vi "uc480_ArrayToImage.vi"(8 "Error In":errorcluster, 10 "InArray":u8[](array[numeric]), 11 ".NET (Reference)":refnum<k24>) -> (0 "Error Out":errorcluster, 2 "Image":picture, 3 "Image Out":T1(plugin-control))   [LabVIEW 2015]
doc: "ArrayToVision converts 24/32-bit one-dimensional arrays to a two-dimensional U32 array."
uses:
  C:/Program Files/Thorlabs/Scientific Imaging/DCx Camera Support/Develop/DotNet/uc480DotNet.dll
  <vilib>/picture/picture.llb/Draw True-Color Pixmap.vi
panel:
  out "SensorColorMode":i32(ring) items=["Invalid"=0, "Monochrome"=1, "Bayer"=2, "CBYCRY"=4, "Jpeg"=8]
  out "Numeric":i32
  # "Input"
  # "Output"
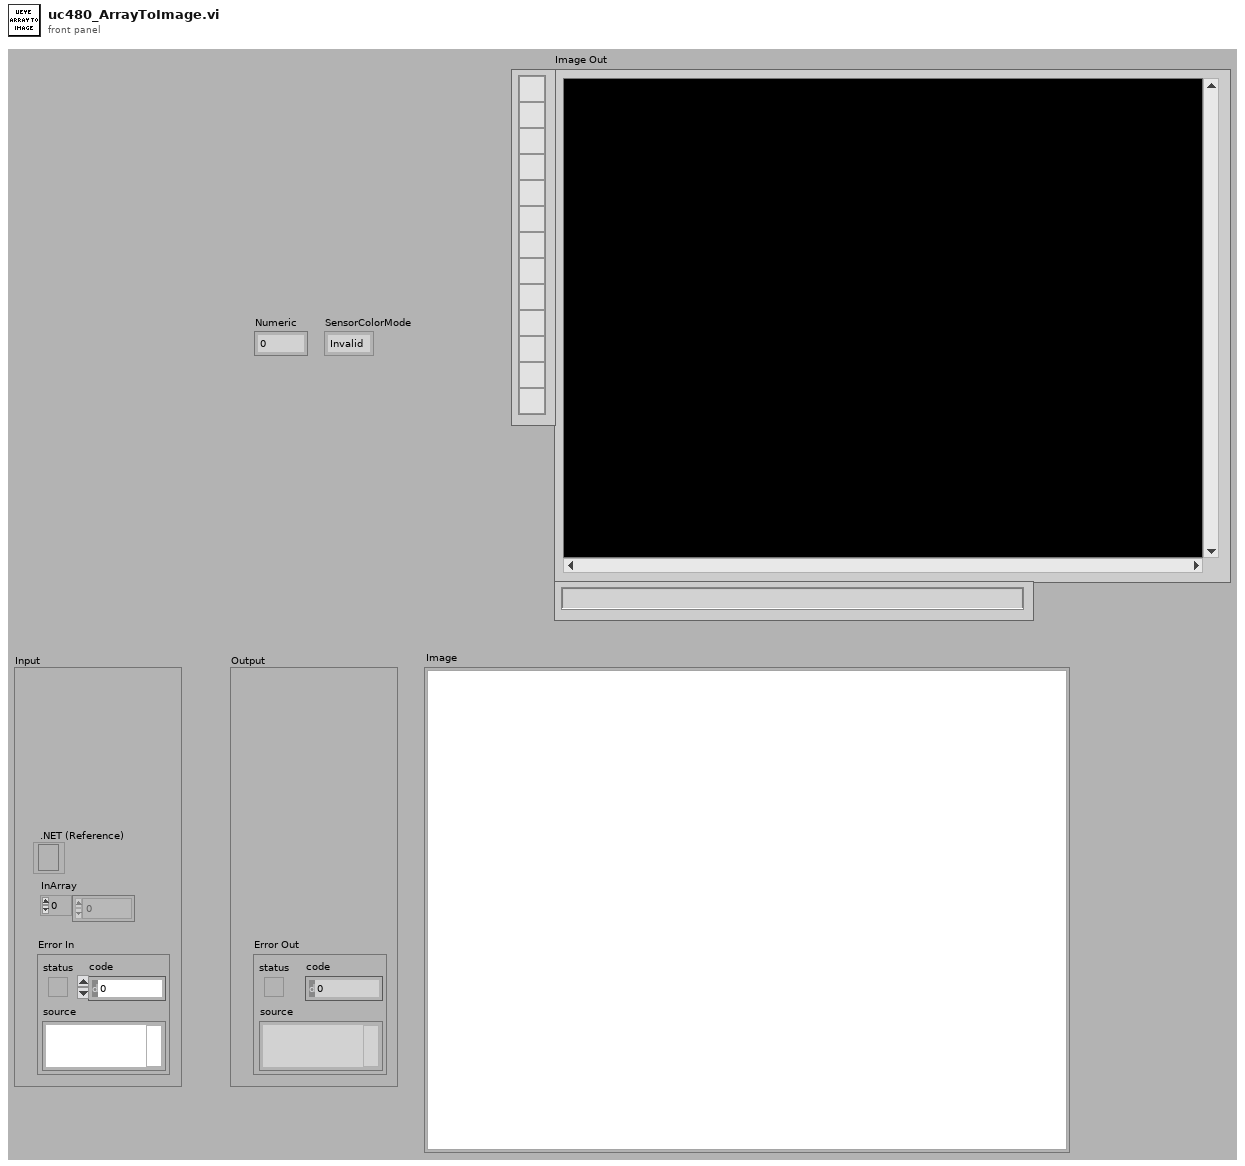
[diagram p1: front panel]
types:
  T1 = typedef "IMAQ Image.ctl" = refnum<image>
  T2 = typedef "Image Type" = u32
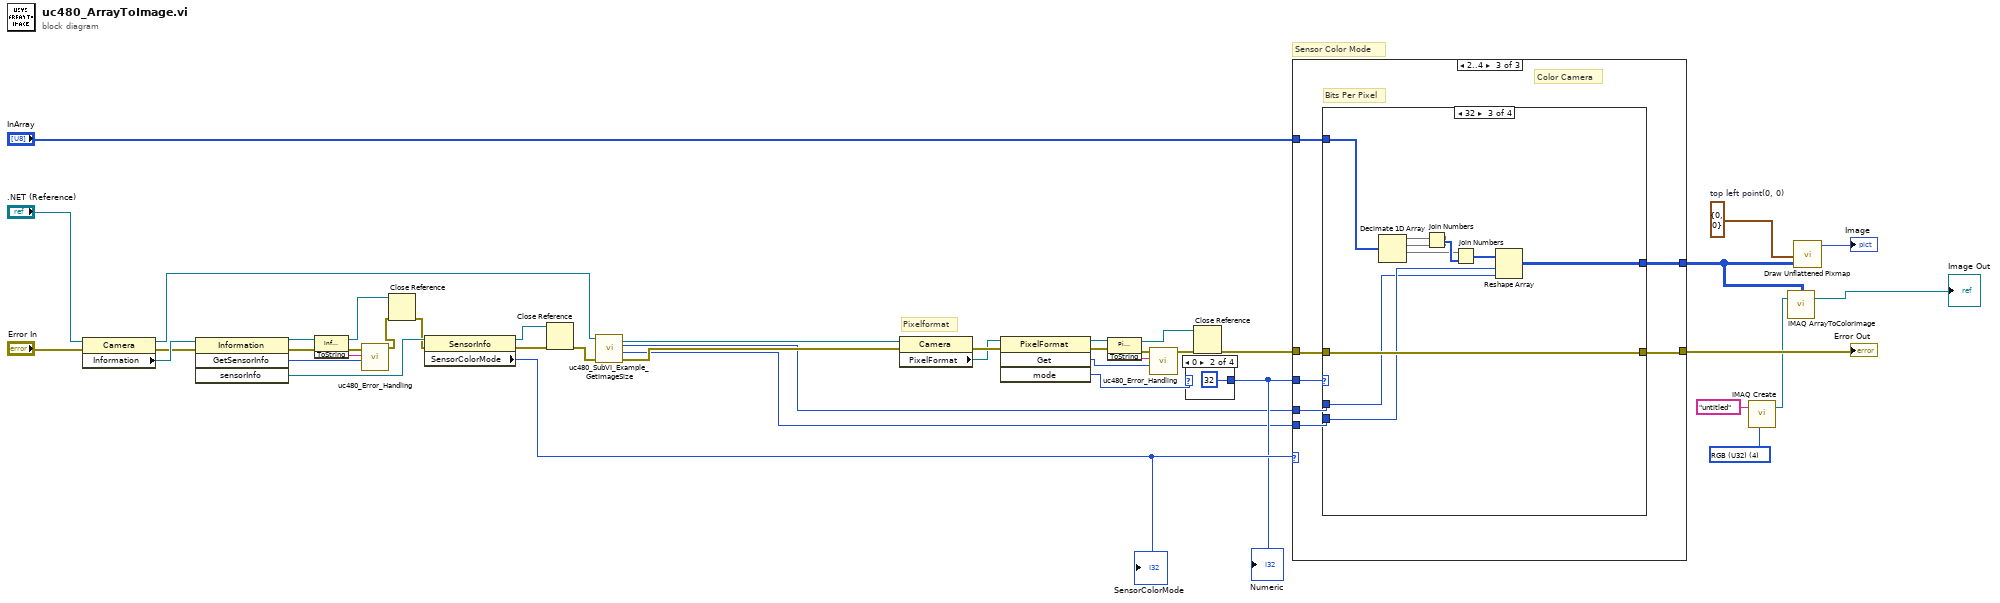
[diagram p0: block diagram]
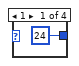
[diagram p2: hidden frame]
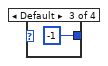
[diagram p3: hidden frame]
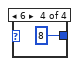
[diagram p4: hidden frame]
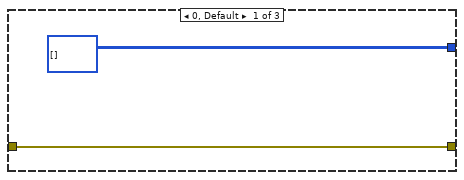
[diagram p5: hidden frame]
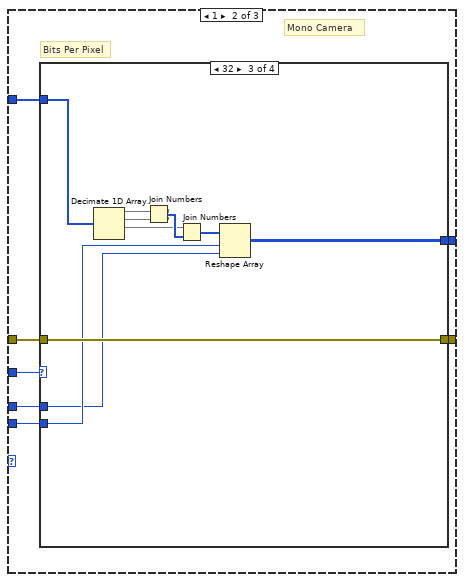
[diagram p6: hidden frame]
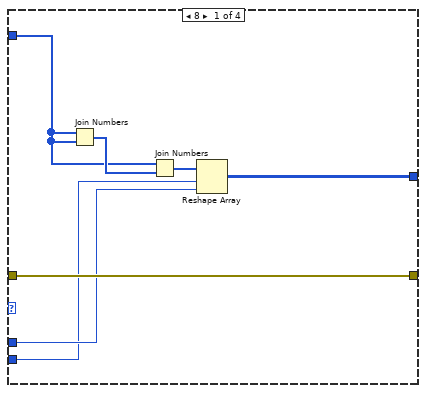
[diagram p7: hidden frame]
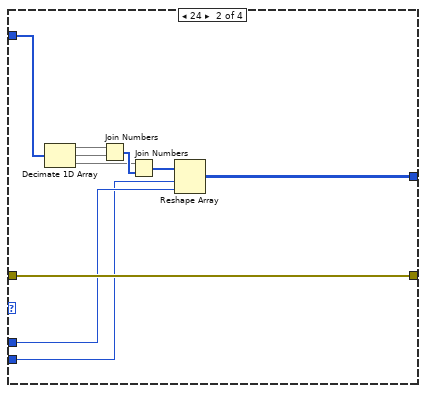
[diagram p8: hidden frame]
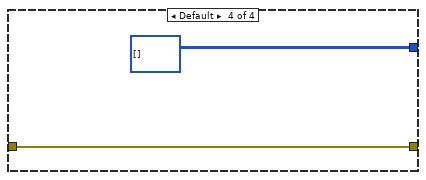
[diagram p9: hidden frame]
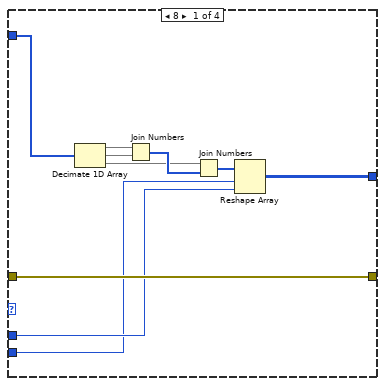
[diagram p10: hidden frame]
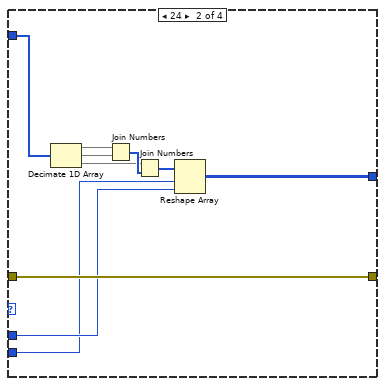
[diagram p11: hidden frame]
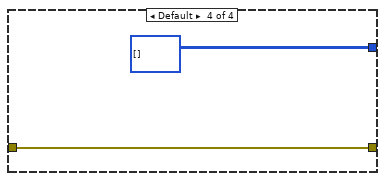
[diagram p12: hidden frame]
diagram:
  w2 = T2 4 items=["Grayscale (U8)", "Grayscale (I16)", "Grayscale (SGL)", "Complex (CSG)", "RGB (U32)", "HSL (U32)", "RGB (U64)", "Grayscale (U16)"] ("Image Type")
  w43 = cluster{i16, i16} {0, 0}  # top left point(0, 0)
  # "Sensor Color Mode"
  # "Pixelformat"
  n1 = property on="Eigenschaftsknoten" class="Camera"(reference=".NET (Reference)", error in="Error In") -> (reference out=w6:refnum<k24>, error out=w38:errorcluster, "Information"=w41:refnum<k24>)
  n2 = invoke class="Information" method="GetSensorInfo"(reference=w41, error in=w38) -> (reference out=w33:refnum<k24>, error out=w32:errorcluster, "GetSensorInfo"=w31:i32, "sensorInfo"=w40:refnum<k24>)  [unwired: 2 in]
  n3 = invoke class="Information" method="ToString"(reference=w33, error in=w32) -> (reference out=w15:refnum<k24>, error out=w35:errorcluster, "ToString"=w34:string)  [unwired: 1 in]
  n4 = call "uc480_Error_Handling.vi"("Error Code"=w31, "Error String"=w34, "Error In"=w35) -> ("Error Out"=w14:errorcluster)  [unwired: 8 in]
  n5 = Close Reference(reference=w15, error in (no error)=w14) -> (error out=w13:errorcluster)
  n6 = property class="SensorInfo"(reference=w40, error in=w13) -> (reference out=w12:refnum<k24>, error out=w11:errorcluster, "SensorColorMode"=w39:i32)
  "SensorColorMode" <- w39
  n7 = Close Reference(reference=w12, error in (no error)=w11) -> (error out=w10:errorcluster)
  n8 = call "uc480_SubVI_Example_GetImageSize.vi"("Error In"=w10, ".NET (Reference)"=w6) -> ("Error Out"=w20:errorcluster, "Height"=w16:i32, "Width"=w17:i32, ".NET (Reference)"=w18:refnum<k24>)  [unwired: 6 in]
  n9 = property class="Camera"(reference=w18, error in=w20) -> (error out=w25:errorcluster, "PixelFormat"=w24:refnum<k24>)  [unwired: 1 out]
  n10 = invoke class="PixelFormat" method="Get"(reference=w24, error in=w25) -> (reference out=w30:refnum<k24>, error out=w29:errorcluster, "Get"=w28:i32, "mode"=w23:i32)  [unwired: 2 in]
  n11 = invoke class="PixelFormat" method="ToString"(reference=w30, error in=w29) -> (reference out=w9:refnum<k24>, error out=w26:errorcluster, "ToString"=w27:string)  [unwired: 1 in]
  n12 = call "uc480_Error_Handling.vi"("Error Code"=w28, "Error String"=w27, "Error In"=w26) -> ("Error Out"=w8:errorcluster)  [unwired: 8 in]
  n13 = case shown="0" w23 {
    tunnel: [24 32 -1 8] -> w22
    frame 1 {
    }
    frame 0 {
    }
    frame Default {
    }
    frame 6 {
    }
  }
  "Numeric" <- w22
  n14 = Close Reference(reference=w9, error in (no error)=w8) -> (error out=w7:errorcluster)
  n15 = case shown="2..4" w39 {
    tunnel: "InArray" -> [_ w53 w92]
    tunnel: w17 -> [_ w51 w87]
    tunnel: w16 -> [_ w50 w86]
    tunnel: w22 -> [_ w52 w88]
    tunnel: w7 -> [w48 w56 w89]
    tunnel: [w48 w55 w90] -> w21
    tunnel: [u32[][] [] w54 w91] -> w1
    frame 0, Default {
    }
    frame 1 {
      # "Bits Per Pixel"
      # "Mono Camera"
      n16 = case shown="32" w52 {
        tunnel: w53 -> [w59 w68 w79 _]
        tunnel: w50 -> [w57 w64 w75 _]
        tunnel: w51 -> [w58 w65 w74 _]
        tunnel: [w63 w67 w81 u32[][] []] -> w54
        tunnel: w56 -> [w62 w66 w80 w84]
        tunnel: [w62 w66 w80 w84] -> w55
        frame 8 {
          n17 = Join Numbers(hi=w59, lo=w59) -> ((hi.lo)=w61:u16[])
          n18 = Join Numbers(hi=w59, lo=w61) -> ((hi.lo)=w60:u32[])
          n19 = Reshape Array(w60, w57, w58) -> (w63:u32[][])
        }
        frame 24 {
          n20 = Decimate 1D Array(w68) -> (w73:u8[], w72:u8[], w70:u8[])
          n21 = Join Numbers(hi=w72, lo=w73) -> ((hi.lo)=w71:u16[])
          n22 = Join Numbers(hi=w70, lo=w71) -> ((hi.lo)=w69:u32[])
          n23 = Reshape Array(w69, w64, w65) -> (w67:u32[][])
        }
        frame 32 {
          n24 = Decimate 1D Array(w79) -> (w78:u8[], w77:u8[], w76:u8[])  [unwired: 1 out]
          n25 = Join Numbers(hi=w77, lo=w78) -> ((hi.lo)=w83:u16[])
          n26 = Join Numbers(hi=w76, lo=w83) -> ((hi.lo)=w82:u32[])
          n27 = Reshape Array(w82, w75, w74) -> (w81:u32[][])
        }
        frame Default {
        }
      }
    }
    frame 2..4 {
      # "Bits Per Pixel"
      # "Color Camera"
      n28 = case shown="32" w88 {
        tunnel: w92 -> [w94 w107 w119 _]
        tunnel: w86 -> [w99 w103 w114 _]
        tunnel: w87 -> [w100 w104 w113 _]
        tunnel: [w102 w106 w120 u32[][] []] -> w91
        tunnel: w89 -> [w101 w105 w118 w123]
        tunnel: [w101 w105 w118 w123] -> w90
        frame 8 {
          n29 = Decimate 1D Array(w94) -> (w98:u8[], w97:u8[], w95:u8[])
          n30 = Join Numbers(hi=w97, lo=w98) -> ((hi.lo)=w96:u16[])
          n31 = Join Numbers(hi=w95, lo=w96) -> ((hi.lo)=w93:u32[])
          n32 = Reshape Array(w93, w99, w100) -> (w102:u32[][])
        }
        frame 24 {
          n33 = Decimate 1D Array(w107) -> (w112:u8[], w111:u8[], w109:u8[])
          n34 = Join Numbers(hi=w111, lo=w112) -> ((hi.lo)=w110:u16[])
          n35 = Join Numbers(hi=w109, lo=w110) -> ((hi.lo)=w108:u32[])
          n36 = Reshape Array(w108, w103, w104) -> (w106:u32[][])
        }
        frame 32 {
          n37 = Decimate 1D Array(w119) -> (w117:u8[], w116:u8[], w115:u8[])  [unwired: 1 out]
          n38 = Join Numbers(hi=w116, lo=w117) -> ((hi.lo)=w122:u16[])
          n39 = Join Numbers(hi=w115, lo=w122) -> ((hi.lo)=w121:u32[])
          n40 = Reshape Array(w121, w114, w113) -> (w120:u32[][])
        }
        frame Default {
        }
      }
    }
  }
  "Error Out" <- w21
  n41 = call "IMAQ Create"("Image Name"="untitled", "Image Type"=w2) -> ("New Image"=w4:T1)  [unwired: 3 in, 1 out]
  n42 = call "IMAQ ArrayToColorImage"("Image Pixels (U32)"=w1, "Image"=w4) -> ("Image Out"=→"Image Out":T1)  [unwired: 3 in, 1 out]
  n43 = call-poly <vilib>:"Draw Unflattened Pixmap.vi"("top left point(0, 0)"=w43, "data (RGB format)"=w1) -> ("new picture"=→"Image":picture)  [unwired: 7 in]
